vi "numbers.vi"() -> ()   [LabVIEW 2013]
uses:
  <vilib>/Utility/file.llb/Read From Spreadsheet File (DBL).vi
panel:
  out "W2/E2":string[](array[string])
  out "W1/E1":string[](array[string])
  out "W/E2":string[](array[string])=["Fore hand", "Back hand", "Over head", "", "Strainght", "Cross", "", "Lob", "Clear", "Drive", "Smash", "Defence", "Chop", "Drop", "Net"]
  out "W/E1":string[](array[string])=["Fore hand", "Back hand", "Over head", "", "Strainght", "Cross", "", "Lob", "Clear", "Drive", "Smash", "Defence", "Chop", "Drop", "Net"]
  out "player2":string[](array[string])
  out "Player 2":string[](array[string])=["Fore hand", "Back hand", "Over head", "", "Strainght", "Cross", "", "Lob", "Clear", "Drive", "Smash", "Defence", "Chop", "Drop", "Net"]
  out "P2graph":cluster{dbl[], "array":dbl[]}(graph)
  out "player2_2":string[](array[string])
  out "p2 6":dbl format="%#.2g"
  out "p2 1":dbl format="%#.2g"
  out "p2 2":dbl format="%#.2g"
  out "p2 3":dbl format="%#.2g"
  out "p2 4":dbl format="%#.2g"
  out "p2 5":dbl format="%#.2g"
  out "p2 7":dbl format="%#.2g"
  out "p2 8":dbl format="%#.2g"
  out "p2 9":dbl format="%#.2g"
  out "p1 9":dbl format="%#.2g"
  out "p1 8":dbl format="%#.2g"
  out "p1 7":dbl format="%#.2g"
  out "p1 6":dbl format="%#.2g"
  out "p1 5":dbl format="%#.2g"
  out "p1 4":dbl format="%#.2g"
  out "p1 3":dbl format="%#.2g"
  out "p1 2":dbl format="%#.2g"
  out "p1 1":dbl format="%#.2g"
  out "player1":string[](array[string])
  out "Player 1":string[](array[string])=["Fore hand", "Back hand", "Over head", "", "Strainght", "Cross", "", "Lob", "Clear", "Drive", "Smash", "Defence", "Chop", "Drop", "Net"]
  out "P1graph":cluster{dbl[], "array":dbl[]}(graph)
  out "player1_2":string[](array[string])
  out "Player 1_2":string[](array[string])=["Fore hand", "Back hand", "Over head", "", "Strainght", "Cross", "", "Lob", "Clear", "Drive", "Smash", "Defence", "Chop", "Drop", "Net"]
  in  "Percentage":bool
  in  "Data file":path caption="Read data from file"
  out "Player 2_2":string[](array[string])=["Fore hand", "Back hand", "Over head", "", "Strainght", "Cross", "", "Lob", "Clear", "Drive", "Smash", "Defence", "Chop", "Drop", "Net"]
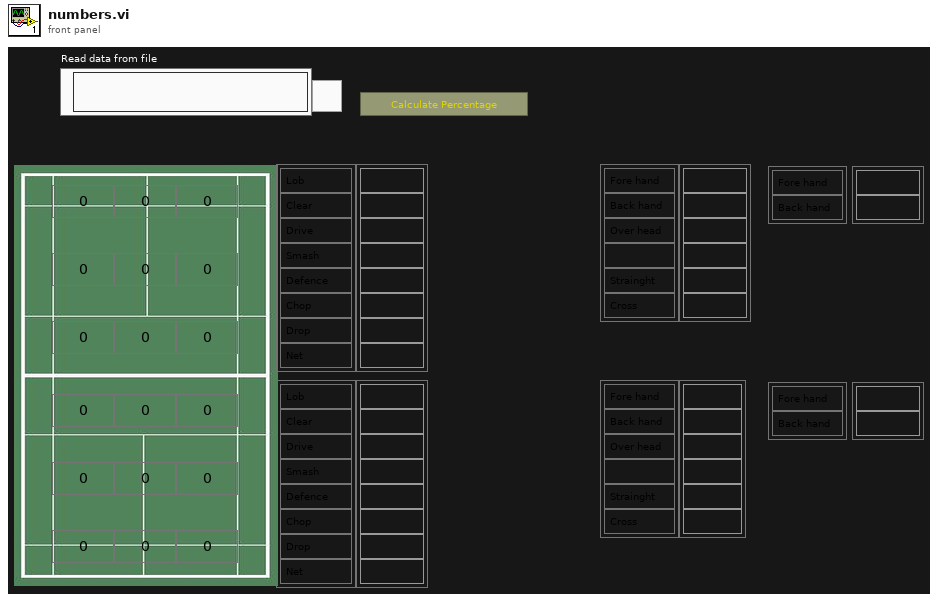
[diagram p1: front panel]
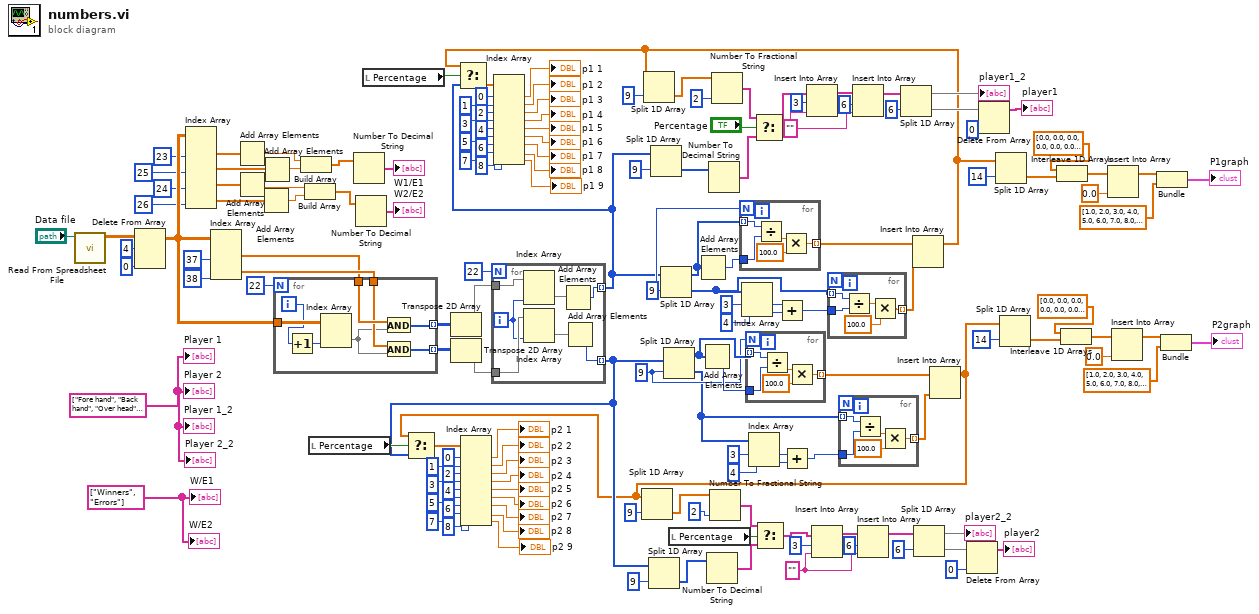
[diagram p0: block diagram]
diagram:
  w28 = string[] ["Winners", "Errors"] ("W/E1")
  w50 = string[] ["Fore hand", "Back hand", "Over head", "", "Strainght", "Cross", "", "Smash", "Defense", "Drive", "Clear", "Drop", "Chop", "Lob", "Net"] ("Player 2")
  w61 = "" ("new element/subarray")
  w62 = "" ("new element/subarray")
  w128 = 9 ("index")
  w133 = 9 ("index")
  n1 = call-poly <vilib>:"Read From Spreadsheet File.vi"("file path (dialog if empty)"="Data file") -> ("all rows"=w150:dbl[][])  [unwired: 6 in, 4 out]
  n2 = Delete From Array(array=w150, length=4, index (row)=0) -> (array with subset deleted=w49:dbl[][])  [unwired: 1 in, 1 out]
  n3 = Index Array(array=w49, index (col) #1=23 ("disabled index (col)"), index (col) #2=25 ("index (col)"), index (col) #3=24 ("index (col)"), index (col) #4=26 ("index (col)")) -> (element #1=w47:dbl[], element #2=w42:dbl[], element #3=w41:dbl[], element #4=w43:dbl[])  [unwired: 4 in]
  n4 = Index Array(array=w49, index (col) #1=37 ("disabled index (col)"), index (col) #2=38 ("index (col)")) -> (element #1=w143:dbl[], element #2=w146:dbl[])  [unwired: 2 in]
  n5 = Add Array Elements(numeric array=w47) -> (sum=w25:dbl)
  n6 = Add Array Elements(numeric array=w41) -> (sum=w26:dbl)
  n7 = Add Array Elements(numeric array=w43) -> (sum=w27:dbl)
  n8 = Add Array Elements(numeric array=w42) -> (sum=w24:dbl)
  n9 = for {
    N: 22 -> [_]
    tunnel: w49 -> [w161]
    tunnel: w143 -> [w160]
    tunnel: w146 -> [w159]
    tunnel: [w157] -> w145 mode=indexing
    tunnel: [w156] -> w144 mode=indexing
    i -> [w154]
    n10 = Increment(x=w154) -> (x+1=w155:i32)
    n11 = Index Array(array=w161, index (col)=w155) -> (element=w158:dbl[])  [unwired: 1 in]
    n12 = And(x=w160, y=w158) -> (x .and. y?=w157:i32[])
    n13 = And(x=w159, y=w158) -> (x .and. y?=w156:i32[])
  }
  n14 = Build Array(w25, w24) -> (w23:dbl[])
  n15 = Build Array(w26, w27) -> (w22:dbl[])
  n16 = local read "Percentage"() -> (w56:bool)
  n17 = Number To Decimal String(number=w23) -> (decimal integer string=→"W1/E1":string[])  [unwired: 1 in]
  n18 = Number To Decimal String(number=w22) -> (decimal integer string=→"W2/E2":string[])  [unwired: 1 in]
  n19 = local read "Percentage"() -> (w53:bool)
  n20 = Transpose 2D Array(2D array=w145) -> (transposed array=w134:i32[][])
  n21 = Transpose 2D Array(2D array=w144) -> (transposed array=w135:i32[][])
  n22 = for {
    N: 22 -> [_]
    tunnel: w134 -> [w168]
    tunnel: w135 -> [w167]
    tunnel: [w164] -> w51 mode=indexing
    tunnel: [w163] -> w55 mode=indexing
    i -> [w166]
    n23 = Index Array(array=w168, index (col)=w166) -> (element=w165:i32[])  [unwired: 1 in]
    n24 = Index Array(array=w167, index (col)=w166) -> (element=w162:i32[])  [unwired: 1 in]
    n25 = Add Array Elements(numeric array=w165) -> (sum=w164:i32)
    n26 = Add Array Elements(numeric array=w162) -> (sum=w163:i32)
  }
  n27 = Split 1D Array(array=w55, index=9) -> (second subarray=w74:i32[])  [unwired: 1 out]
  n28 = Split 1D Array(array=w51, index=9) -> (second subarray=w80:i32[])  [unwired: 1 out]
  n29 = Split 1D Array(array=w51, index=w133) -> (first subarray=w132:i32[], second subarray=w122:i32[])
  n30 = Split 1D Array(array=w55, index=w128) -> (first subarray=w129:i32[], second subarray=w124:i32[])
  n31 = local read "Percentage"() -> (w70:bool)
  n32 = Add Array Elements(numeric array=w132) -> (sum=w131:i32)
  n33 = Add Array Elements(numeric array=w129) -> (sum=w130:i32)
  n34 = Number To Decimal String(number=w74) -> (decimal integer string=w68:string[])  [unwired: 1 in]
  n35 = Number To Decimal String(number=w80) -> (decimal integer string=w71:string[])  [unwired: 1 in]
  n36 = for {
    N: w133 -> [_]
    tunnel: w132 -> [w173] mode=indexing
    tunnel: w131 -> [w172]
    tunnel: [w169] -> w87 mode=indexing
    n37 = Divide(x=w173, y=w172) -> (x/y=w171:dbl)
    n38 = Multiply(x=w171, y=100.0) -> (x*y=w169:dbl)
  }
  n39 = Index Array(array=w122, index #1=3 ("index"), index #2=4 ("index")) -> (element #1=w127:i32, element #2=w126:i32)
  n40 = for {
    N: w128 -> [_]
    tunnel: w129 -> [w178] mode=indexing
    tunnel: w130 -> [w177]
    tunnel: [w174] -> w85 mode=indexing
    n41 = Divide(x=w178, y=w177) -> (x/y=w176:dbl)
    n42 = Multiply(x=w176, y=100.0) -> (x*y=w174:dbl)
  }
  n43 = Index Array(array=w124, index #1=3 ("index"), index #2=4 ("index")) -> (element #1=w136:i32, element #2=w137:i32)
  n44 = Add(x=w127, y=w126) -> (x+y=w123:i32)
  n45 = Add(x=w136, y=w137) -> (x+y=w125:i32)
  n46 = for {
    tunnel: w122 -> [w183] mode=indexing
    tunnel: w123 -> [w182]
    tunnel: [w179] -> w86 mode=indexing
    n47 = Divide(x=w183, y=w182) -> (x/y=w181:dbl)
    n48 = Multiply(x=w181, y=100.0) -> (x*y=w179:dbl)
  }
  n49 = for {
    tunnel: w124 -> [w188] mode=indexing
    tunnel: w125 -> [w187]
    tunnel: [w184] -> w84 mode=indexing
    n50 = Divide(x=w188, y=w187) -> (x/y=w186:dbl)
    n51 = Multiply(x=w186, y=100.0) -> (x*y=w184:dbl)
  }
  n52 = Insert Into Array(array=w87, new element=w86) -> (w18:dbl[])  [unwired: 1 in]
  n53 = Select(t=w18, s=w53, f=w51) -> (s? t:f=w52:dbl[])
  n54 = Index Array(array=w52, index #1=0 ("index"), index #2=1 ("index"), index #3=2 ("index"), index #4=3 ("index"), index #5=4 ("index"), index #6=5 ("index"), index #7=6 ("index"), index #8=7 ("index"), index #9=8 ("index")) -> (element #1=→"p1 1":dbl, element #2=→"p1 2":dbl, element #3=→"p1 3":dbl, element #4=→"p1 4":dbl, element #5=→"p1 5":dbl, element #6=→"p1 6":dbl, element #7=→"p1 7":dbl, element #8=→"p1 8":dbl, element #9=→"p1 9":dbl)
  n55 = Split 1D Array(array=w18, index=9) -> (second subarray=w78:dbl[])  [unwired: 1 out]
  n56 = Number To Fractional String(number=w78, precision (6)=i16 2) -> (F-format string=w72:string[])  [unwired: 2 in]
  n57 = Select(t=w72, s="Percentage", f=w71) -> (s? t:f=w66:string[])
  n58 = Insert Into Array(array=w66, index=3, new element=w62) -> (w64:string[])
  n59 = Insert Into Array(array=w64, index=6, new element=w62) -> (w39:string[])
  n60 = Split 1D Array(array=w39, index=6) -> (first subarray=→"player1_2":string[], second subarray=w36:string[])
  n61 = Insert Into Array(array=w85, new element=w84) -> (w2:dbl[])  [unwired: 1 in]
  n62 = Select(t=w2, s=w56, f=w55) -> (s? t:f=w54:dbl[])
  n63 = Index Array(array=w54, index #1=0 ("index"), index #2=1 ("index"), index #3=2 ("index"), index #4=3 ("index"), index #5=4 ("index"), index #6=5 ("index"), index #7=6 ("index"), index #8=7 ("index"), index #9=8 ("index")) -> (element #1=→"p2 1":dbl, element #2=→"p2 2":dbl, element #3=→"p2 3":dbl, element #4=→"p2 4":dbl, element #5=→"p2 5":dbl, element #6=→"p2 6":dbl, element #7=→"p2 7":dbl, element #8=→"p2 8":dbl, element #9=→"p2 9":dbl)
  n64 = Split 1D Array(array=w2, index=9) -> (second subarray=w77:dbl[])  [unwired: 1 out]
  n65 = Number To Fractional String(number=w77, precision (6)=i16 2) -> (F-format string=w69:string[])  [unwired: 2 in]
  n66 = Select(t=w69, s=w70, f=w68) -> (s? t:f=w57:string[])
  n67 = Insert Into Array(array=w57, index=3, new element=w61) -> (w59:string[])
  n68 = Insert Into Array(array=w59, index=6, new element=w61) -> (w31:string[])
  n69 = Split 1D Array(array=w31, index=6) -> (first subarray=→"player2_2":string[], second subarray=w33:string[])
  n70 = Delete From Array(array=w33, index=0) -> (array with subset deleted=→"player2":string[])  [unwired: 1 in, 1 out]
  n71 = Delete From Array(array=w36, index=0) -> (array with subset deleted=→"player1":string[])  [unwired: 1 in, 1 out]
  n72 = Split 1D Array(array=w18, index=14) -> (second subarray=w16:dbl[])  [unwired: 1 out]
  n73 = Split 1D Array(array=w2, index=14) -> (second subarray=w5:dbl[])  [unwired: 1 out]
  n74 = Interleave 1D Arrays(dbl[] [0.0, 0.0, 0.0, 0.0, 0.0, 0.0, 0.0, 0.0] ("array"), w16) -> (w13:dbl[])
  n75 = Interleave 1D Arrays(dbl[] [0.0, 0.0, 0.0, 0.0, 0.0, 0.0, 0.0, 0.0] ("array"), w5) -> (w8:dbl[])
  n76 = Insert Into Array(array=w13, new element=0.0 ("new element/subarray")) -> (w11:dbl[])  [unwired: 1 in]
  n77 = Insert Into Array(array=w8, new element=0.0 ("new element/subarray")) -> (w10:dbl[])  [unwired: 1 in]
  n78 = Bundle(w11, "array"=dbl[] [1.0, 2.0, 3.0, 4.0, 5.0, 6.0, 7.0, 8.0, 9.0, 10.0, 11.0, 12.0, 13.0, 14.0, 15.0, 16.0, 17.0]) -> (→"P1graph":cluster{dbl[], "array":dbl[]})  [unwired: 1 in]
  n79 = Bundle(w10, "array"=dbl[] [1.0, 2.0, 3.0, 4.0, 5.0, 6.0, 7.0, 8.0, 9.0, 10.0, 11.0, 12.0, 13.0, 14.0, 15.0, 16.0, 17.0]) -> (→"P2graph":cluster{dbl[], "array":dbl[]})  [unwired: 1 in]
  "Player 1" <- w50
  "Player 1_2" <- w50
  "Player 2_2" <- w50
  "Player 2" <- w50
  "W/E1" <- w28
  "W/E2" <- w28
